vi "array_calc.vi"() -> ()   [LabVIEW 2013]
panel:
  in  "stop":bool
  in  "sortowanie":enum16{"rosnaco", "malejaco"}(ring)
  out "posortowane":dbl[](array[numeric])
  out "srednia":dbl
  out "min value":dbl
  out "max value":dbl
  in  "wejscie":dbl[](array[numeric])
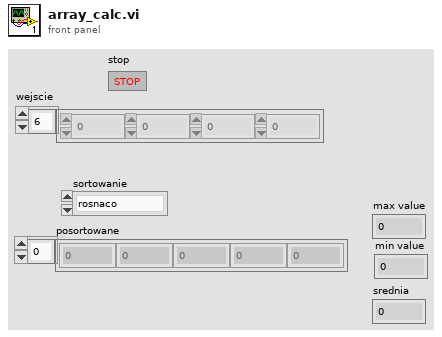
[diagram p1: front panel]
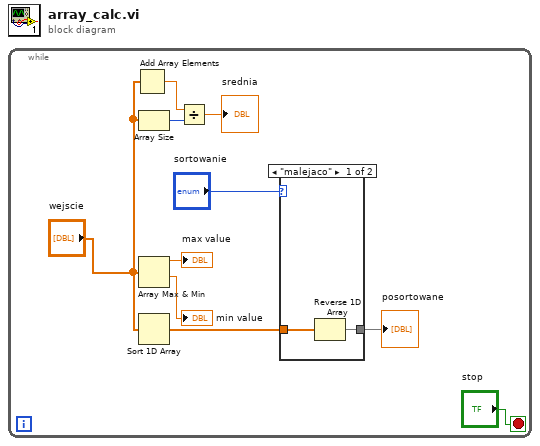
[diagram p0: block diagram]
diagram:
  n1 = while {
    stop <- "stop" stop-if-true
    n2 = Add Array Elements(numeric array="wejscie") -> (sum=w8:dbl)
    n3 = Array Size(array="wejscie") -> (size(s)=w6:i32)
    n4 = Array Max & Min(array="wejscie") -> (max value=→"max value":dbl, min value=→"min value":dbl)  [unwired: 2 out]
    n5 = Sort 1D Array(array="wejscie") -> (sorted array=w5:dbl[])
    n6 = Divide(x=w8, y=w6) -> (x/y=→"srednia":dbl)
    n7 = case shown="\"malejaco\"" "sortowanie" {
      tunnel: w5 -> [w12 w13]
      tunnel: [w11 w13] -> w3
      frame "malejaco" {
        n8 = Reverse 1D Array(array=w12) -> (reversed array=w11:dbl[])
      }
      frame "rosnaco", Default {
      }
    }
    "posortowane" <- w3
  }
